vi "Build Installer.vi"(8 "error in (no error)":errorcluster, 11 "PostBuildSupport in":refnum<class "PostBuildSupport.lvclass">) -> (0 "error out":errorcluster, 3 "PostBuildSupport out":refnum<class "PostBuildSupport.lvclass">)   [LabVIEW 2016, in "PostBuildSupport.lvclass"]
uses:
  PostBuildSupport.lvclass
  PostBuildSupport.lvclass/PostBuildSupport.ctl
  <vilib>/AppBuilder/AB_API_Simple/Build (path).vi
  <vilib>/AppBuilder/AB_API_Simple/NI_App_Builder_API.lvlib
panel:
  out "Progress Bar":u8(slide) caption="Opening PPMS Monitor and Control Installer" scale=0.0..100.0
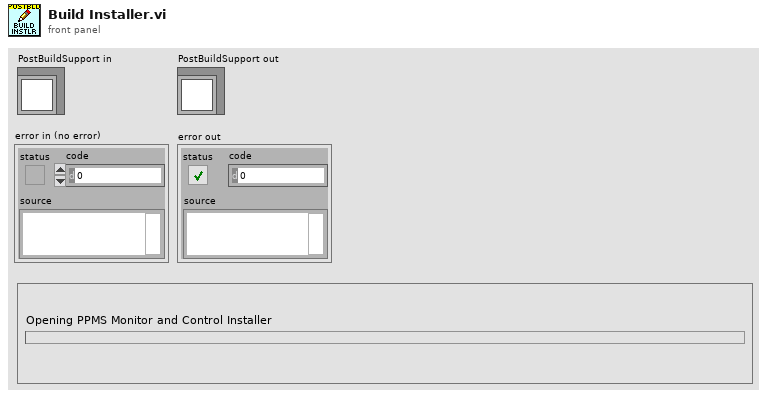
[diagram p1: front panel]
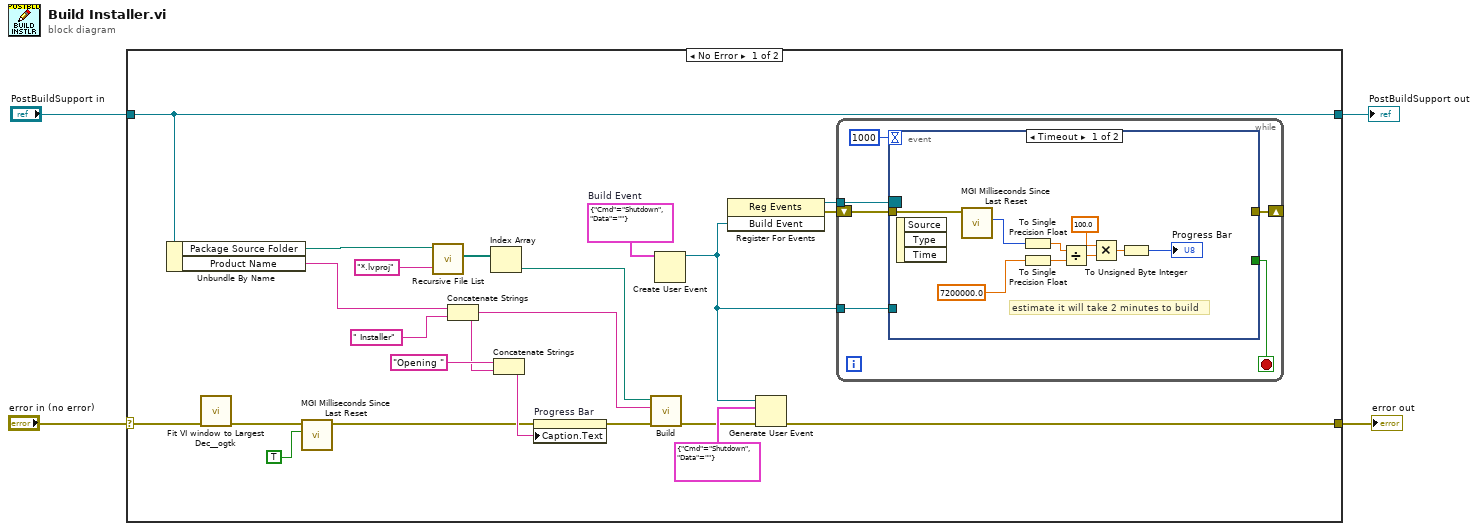
[diagram p0: block diagram]
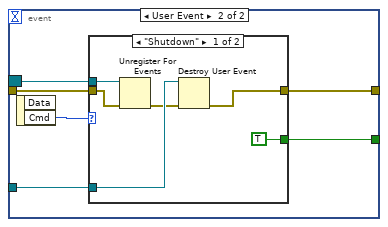
[diagram p2: hidden frame]
diagram:
  n1 = case shown="No Error" "error in (no error)" {
    selector: "error in (no error)" -> [w20 w56]
    tunnel: "PostBuildSupport in" -> [w22 w55]
    tunnel: [w8 w56] -> w2
    tunnel: [w22 w55] -> w1
    frame No Error {
      w14 = cluster{"Cmd":enum16{"Shutdown"}, "Data":string} {"Cmd"=enum."Shutdown", "Data"=""}  # Build Event
      n2 = Unbundle By Name(w22) -> ("Package Source Folder"=w19:path, "Product Name"=w23:string)
      n3 = call <userlib>:"Fit VI window to Largest Dec__ogtk.vi"("error in (no error)"=w20) -> ("error out"=w6:errorcluster)  [unwired: 5 in, 1 out]
      n4 = call <userlib>:"MGI Milliseconds Since Last Reset.vi"("Reset (F)"=TRUE, "Error In"=w6) -> ("Error Out"=w5:errorcluster)  [unwired: 4 in, 1 out]
      n5 = call <vilib>:"Recursive File List.vi"("pattern"="*.lvproj", "Folder Path"=w19) -> ("All Files in Dir"=w24:path[])  [unwired: 5 in, 4 out]
      n6 = Concatenate Strings(w23, " Installer" ("Name of target (My Computer)")) -> (w16:string)
      n7 = Index Array(array=w24) -> (element=w15:path)  [unwired: 1 in]
      n8 = Concatenate Strings("Opening " ("string"), w16) -> (w18:string)
      n9 = property on="Progress Bar" class="Slide (strict)"(error in=w5, "Caption.Text"=w18) -> (error out=w17:errorcluster)  [unwired: 1 in, 1 out]
      n10 = call-poly <vilib>:"Build.vi"("error in (no error)"=w17, "Name of build specification (if empty: build all)"=w16, "Path to project"=w15) -> ("error out"=w12:errorcluster)  [unwired: 7 in, 1 out]
      n11 = Create User Event(user event datatype=w14) -> (user event=w10:refnum<user-event>)  [unwired: 1 in, 1 out]
      n12 = register-events(w10) -> (reference out=w11:refnum<event-registration>, error out=w9:errorcluster)  [unwired: 2 in]
      n13 = Generate User Event(user event=w10, event data cluster=cluster{"Cmd":enum16{"Shutdown"}, "Data":string} {"Cmd"=enum."Shutdown", "Data"=""} ("event data"), error in=w12) -> (error out=w8:errorcluster)  [unwired: 1 in, 1 out]
      n14 = while {
        tunnel: w11 -> [w32]
        tunnel: w10 -> [w31]
        shift-right: [w29] -> _
        shift-left: w9 -> [w30]
        stop <- w28 stop-if-true
        n15 = event shown="[0] Timeout" {
          selector: w32 -> [_ w45]
          dyn-events: _ -> [_ _]
          timeout: 1000 -> [_ _]
          tunnel: w31 -> [_ w47]
          tunnel: w30 -> [w35 w46]
          tunnel: [_ w44] -> w29
          tunnel: [_ w43] -> w28
          event Timeout {
            # "estimate it will take 2 minutes to build"
            n16 = event-data() -> ()  [unwired: 1 in, 3 out]
            n17 = call <userlib>:"MGI Milliseconds Since Last Reset.vi"("Error In"=w35) -> ("ms"=w34:u32)  [unwired: 5 in, 1 out]
            n18 = To Single Precision Float(number=w34) -> (single precision float=w38:sgl)
            n19 = To Single Precision Float(number=sgl 7200000.0) -> (single precision float=w37:sgl)
            n20 = Divide(x=w38, y=w37) -> (x/y=w39:sgl)
            n21 = Multiply(x=sgl 100.0, y=w39) -> (x*y=w41:sgl)
            n22 = To Unsigned Byte Integer(number=w41) -> (unsigned 8bit integer=→"Progress Bar":u8)
          }
          event User Event {
            n23 = event-data() -> ("Cmd"=w42:enum16{"Shutdown"})  [unwired: 1 in, 1 out]
            n24 = case shown="\"Shutdown\"" w42 {
              tunnel: [TRUE _] -> w43
              tunnel: w45 -> [w52 _]
              tunnel: [w48 w54] -> w44
              tunnel: w46 -> [w51 w54]
              tunnel: w47 -> [w50 _]
              frame "Shutdown" {
                n25 = Unregister For Events(event registration refnum=w52, error in=w51) -> (error out=w49:errorcluster)
                n26 = Destroy User Event(user event=w50, error in=w49) -> (error out=w48:errorcluster)
              }
              frame Default {
              }
            }
          }
        }
      }
    }
    frame Error {
    }
  }
  "error out" <- w2
  "PostBuildSupport out" <- w1
